vi "ADC SNR_Sweep_working.vi"(8 "error in (no error)":errorcluster, 9 "Sequence parameters":string[][](array[string])=[["Min limit", "Max limit", "Register sheet file", "Register Sheet"], ["", "", "CC2600.xls", "TX_BLE;Trim"], ["Reg write (addr;value)", "Operating frequency [Hz]", "", ""], ["NA", "2.44G", "", ""]], 10 "Run type":i32, 11 "Method parameters":T3={"Dev"={"Do not disturb DUT"=FALSE, "XOSC"=32000000.0, "Board type"="", "EM"="", "Configure tempboard"=TRUE, "Device specific info"=[], "Generic Object"=refnum}, "Method"={"Run type"=1, "Test name"="Current LPM2 4", "Comment"="", "Results folder"="", "AFC"=enum."Off", "Method name"="Current LPM2 4", "Method results"={"Excel brief report"=FALSE, "Spotfire report"=FALSE, "Starfish report"=FALSE}, "Operator"="", "Reference time"=timestamp(0 s since 1904-01-01), "AFC delay"=0.0, "Initialization"=enum."Enabled", "MD5 Sum"="", "HW addon board"=enum."None", "AFC Regsheet"="", "AFC Regfile"=path "", "dummy"=0.0}, "Inst"={"Instr"={"PS1"={"Name"="", "GPIB address"="", "VISA session"=""}, "PS2"={"Name"="", "GPIB address"="", "VISA session"=""}, "TC1"={"Name"="", "GPIB address"="", "VISA session"=""}, "TC2"={"Name"="", "GPIB address"="", "VISA session"=""}, "SA1"={"Name"="", "GPIB address"="", "VISA session"=""}, "SA2"={"Name"="", "GPIB address"="", "VISA session"=""}, "SG1"={"Name"="", "GPIB address"="", "VISA session"=""}, "SG2"={"Name"="", "GPIB address"="", "VISA session"=""}, "SG3"={"Name"="", "GPIB address"="", "VISA session"=""}, "MI1"={"Name"="", "GPIB address"="", "VISA session"=""}, "MI2"={"Name"="", "GPIB address"="", "VISA session"=""}, "SW SA"={"Name"="", "Controller addr"=""}, "SW SG"={"Name"="", "Controller addr"=""}, "MI3"={"Name"="", "GPIB address"="", "VISA session"=""}}, "Switchbox"={"RF Path"=0, "Cal compensation"=enum."TX", "Switchbox gain mode"="", "State"=enum."TX"}, "Instr to control (i.e. SA1)"="Default", "Intrument info string"=""}, "Sequence parameters"=[["Weight", "Min Limit", "Max Limit", "Register Sheet", "", "", "", "", "", "", "", "", ""], ["Vital", "", "1", "LPM2", "", "", "", "", "", "", "", "", ""], ["Resolution", "Reg write (addr;value)", "Chip mode", "Range", "", "", "", "", "", "", "", "", ""], ["u", "NA", "", "auto", "", "", "", "", "", "", "", "", ""]], "Cond"={"Temp logged"=25.0, "VDD1_PS1_6V"=-999.0, "VDD2_PS1_25V"=-999.0, "VDD4_PS2_25V"=-999.0, "VDD3_PS2_6V"=-999.0}, "Meas config"={"X-axis inner loop index"=32000000, "Y-axis outer loop index"=32000000, "X-axis"=[], "Y-axis"=[], "X-axis array req size"=32000000, "Y-axis array req size"=32000000, "Param description"=[], "Use meas clust for reporting"=FALSE, "Parameter index (page)"=0, "X-axis name"="", "Y-axis name"=""}} {"Cond"."VDD3_PS2_6V" format="%.3f"; "Cond"."VDD4_PS2_25V" format="%.3f"; "Cond"."VDD2_PS1_25V" format="%.3f"; "Cond"."VDD1_PS1_6V" format="%.3f"; "Method"."dummy" format="%.1p"; "Method"."AFC delay" format="%.1p"; "Dev"."XOSC" format="%.3p"}) -> (0 "error out":errorcluster, 1 "End method error":T1, 2 "Short Results":string[](array[string]), 3 "Result summary":string[][](array[string])=[["Critical", "Output Power@2405 MHz", "-3", "4", "dBm"], ["Critical", "Output Power@2410 MHz", "-3", "4", "dBm"]])   [LabVIEW 2019]
doc: "[AutoDocStart]Performs crystal accuracy measurements. Measures the offset from ideal frequency. Primarily used for tuning XOSC capacitors and verifying XOSC trims.\n\nSweeping parameters: operating frequency, OSC override value and VDDR level\n\nResults: Offset frequency in ppm[AutoDocEnd]"
uses:
  User Lib/Utilities/Cluster definitions/Method input.ctl
  User Lib/Utilities/Cluster definitions/Device specific info.ctl
  User Lib/Utilities/Controls/Automatic Frequency Compensation types.ctl
  User Lib/Utilities/Controls/Method Reports.ctl
  User Lib/Utilities/Cluster definitions/Method Initialization.ctl
  User Lib/Utilities/Controls/HW addon boards.ctl
  User Lib/Utilities/Cluster definitions/Instr clust.ctl
  User Lib/Utilities/Switchbox control/SwitchBox_State._ENUMctl.ctl
  User Lib/Utilities/Cluster definitions/End method error cluster.ctl
  669fe48b-0ce9-4029-a6ff-6e407436e5b7.vi
  160c279e-5860-4c4e-a522-43dd8a66307b.vi
  470ab757-4a27-4988-8e62-97c7fe5a2084.vi
  56529db9-b118-41d0-9f0e-72512248274d.vi
panel:
  in  "Tab Control":T2(tab)
  # "°C"
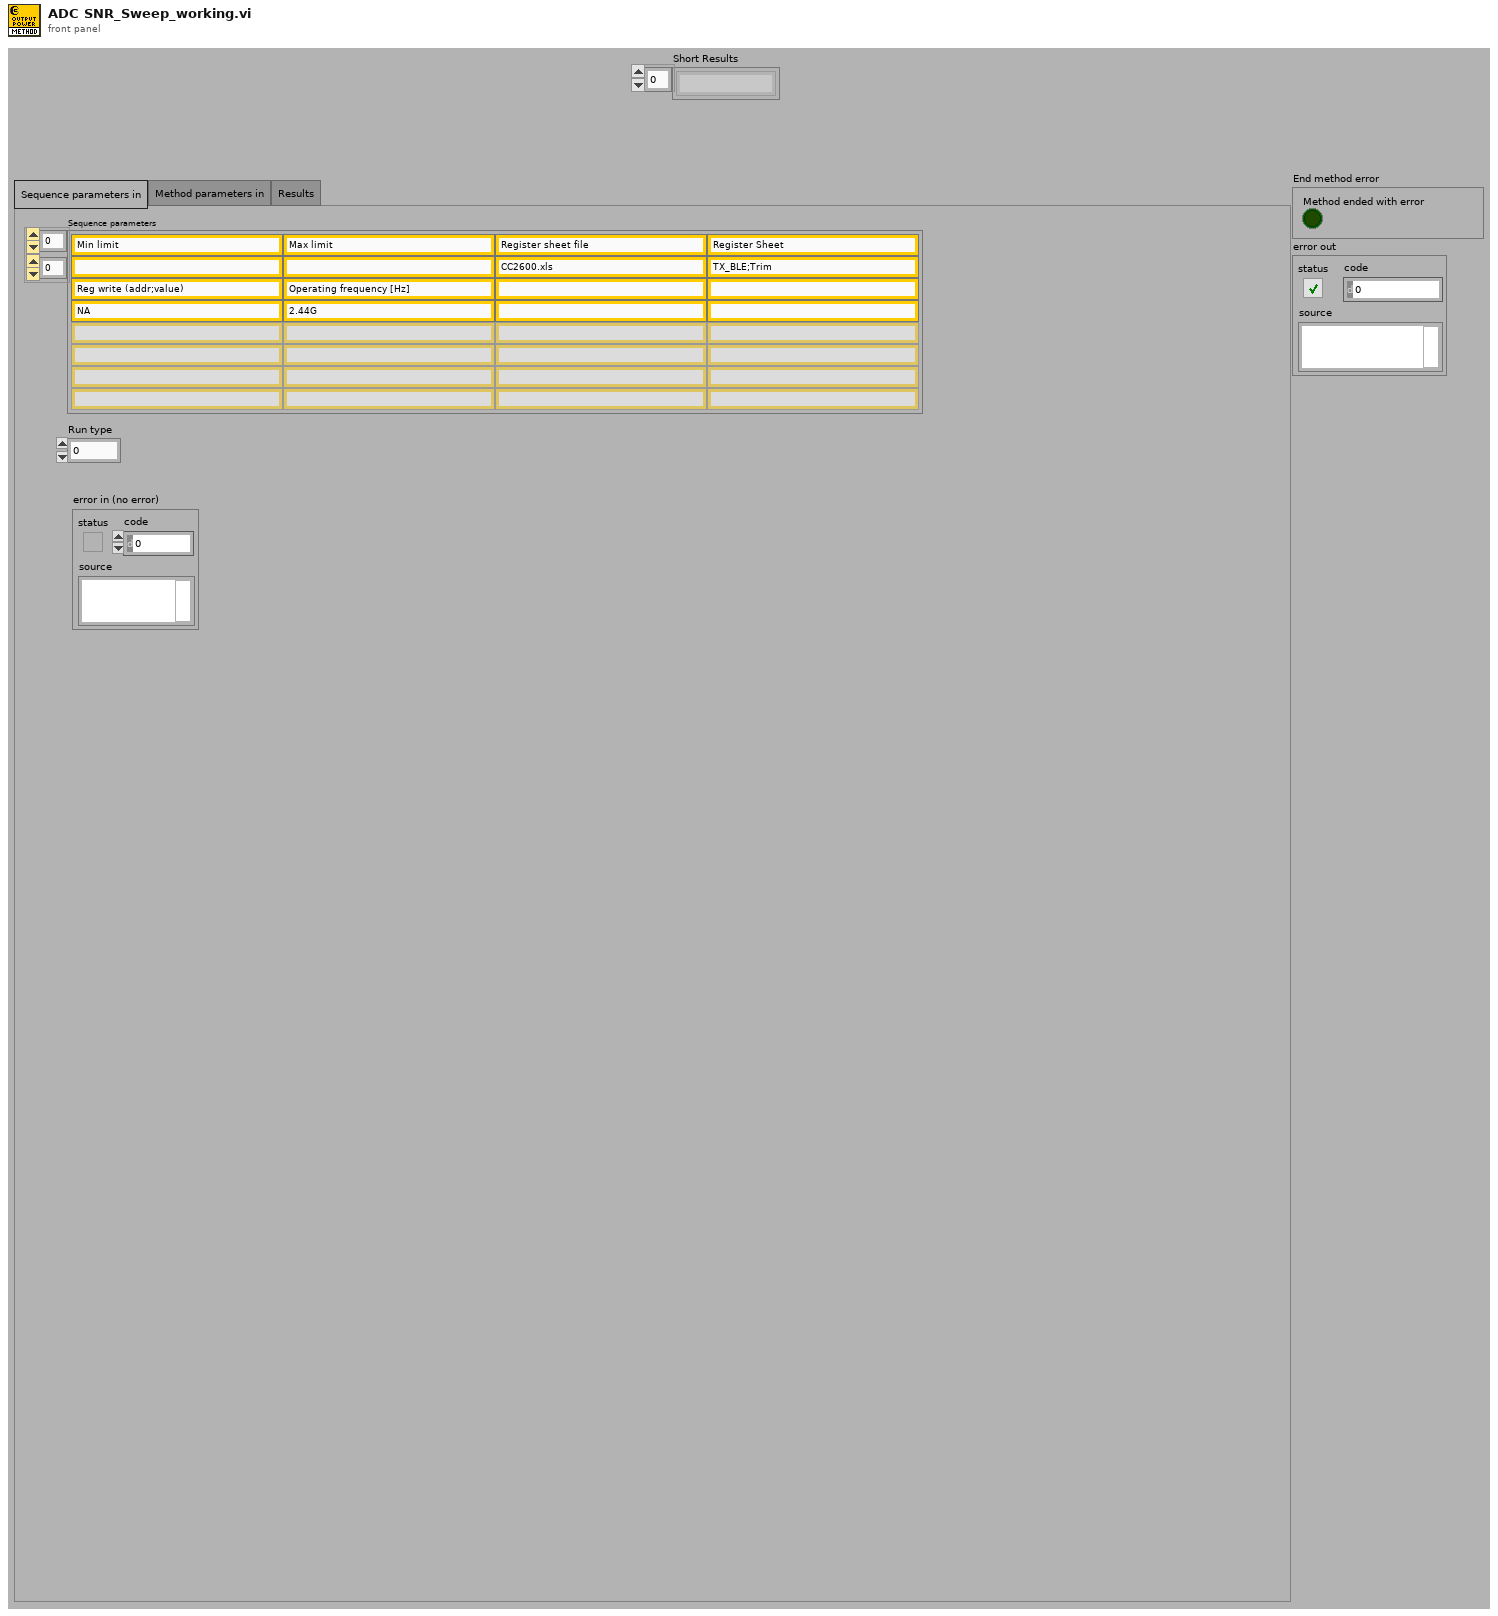
[diagram p1: front panel]
types:
  T1 = typedef "End method error cluster.ctl" = cluster{"Method ended with error":bool}
  T2 = enum32{"Sequence parameters in", "Method parameters in", "Results"}
  T3 = typedef "Method input.ctl" = cluster{"Dev":cluster{"Do not disturb DUT":bool, "XOSC":dbl, "Board type":string, "EM":string, "Configure tempboard":bool, "Device specific info":T4[], "Generic Object":refnum<class>}, "Method":cluster{"Run type":i32, "Test name":string, "Comment":string, "Results folder":string, "AFC":T5, "Method name":string, "Method results":T6, "Operator":string, "Reference time":timestamp, "AFC delay":dbl, "Initialization":T7, "MD5 Sum":string, "HW addon board":T8, "AFC Regsheet":string, "AFC Regfile":path, "dummy":dbl}, "Inst":T9, "Sequence parameters":string[][], "Cond":cluster{"Temp logged":dbl, "VDD1_PS1_6V":dbl, "VDD2_PS1_25V":dbl, "VDD4_PS2_25V":dbl, "VDD3_PS2_6V":dbl}, "Meas config":cluster{"X-axis inner loop index":i32, "Y-axis outer loop index":i32, "X-axis":string[], "Y-axis":string[], "X-axis array req size":i32, "Y-axis array req size":i32, "Param description":string[][], "Use meas clust for reporting":bool, "Parameter index (page)":i32, "X-axis name":string, "Y-axis name":string}}
  T4 = typedef "Device specific info.ctl" = cluster{"EM number":u8, "IP address":string, "Enabled":bool, "Slot no":u8, "RF path":u8, "EM name":string, "Wafer info":string, "AFC frequency ppm":dbl, "Register writes":string[][], "Meas data":string[][][], "Device comment":string}
  T5 = typedef "Automatic Frequency Compensation types.ctl" = enum16{"Off", "Compensate Instrument frequency", "Compensate DUT frequency", "Predictive - Compensate Instrument frequency", "Predictive - Compensate DUT frequency", "Do not skip re-init - Compensate Instrument frequency", "Do not skip re-init - Compensate DUT frequency"}
  T6 = typedef "Method Reports.ctl" = cluster{"Excel brief report":bool, "Spotfire report":bool, "Starfish report":bool}
  T7 = typedef "Method Initialization.ctl" = enum16{"Enabled", "Skip Instr and Device Init", "Enabled with Separate Flash", "Set PS, Device Init and Skip Instr Init", "Skip Device Init"}
  T8 = typedef "HW addon boards.ctl" = enum16{"None", "Current meas 5EM", "Stresstest 10EM"}
  T9 = typedef "Instr clust.ctl" = cluster{"Instr":cluster{"PS1":cluster{"Name":string, "GPIB address":string, "VISA session":refnum<visa-resource-name>}, "PS2":cluster{"Name":string, "GPIB address":string, "VISA session":refnum<visa-resource-name>}, "TC1":cluster{"Name":string, "GPIB address":string, "VISA session":refnum<visa-resource-name>}, "TC2":cluster{"Name":string, "GPIB address":string, "VISA session":refnum<visa-resource-name>}, "SA1":cluster{"Name":string, "GPIB address":string, "VISA session":refnum<visa-resource-name>}, "SA2":cluster{"Name":string, "GPIB address":string, "VISA session":refnum<visa-resource-name>}, "SG1":cluster{"Name":string, "GPIB address":string, "VISA session":refnum<visa-resource-name>}, "SG2":cluster{"Name":string, "GPIB address":string, "VISA session":refnum<visa-resource-name>}, "SG3":cluster{"Name":string, "GPIB address":string, "VISA session":refnum<visa-resource-name>}, "MI1":cluster{"Name":string, "GPIB address":string, "VISA session":refnum<visa-resource-name>}, "MI2":cluster{"Name":string, "GPIB address":string, "VISA session":refnum<visa-resource-name>}, "SW SA":cluster{"Name":string, "Controller addr":string}, "SW SG":cluster{"Name":string, "Controller addr":string}, "MI3":cluster{"Name":string, "GPIB address":string, "VISA session":refnum<visa-resource-name>}}, "Switchbox":cluster{"RF Path":i32, "Cal compensation":enum16{"TX", "RX", "Interferer", "No compensation", "Interferer2"}, "Switchbox gain mode":string, "State":T10}, "Instr to control (i.e. SA1)":string, "Intrument info string":string}
  T10 = typedef "SwitchBox_State._ENUMctl.ctl" = enum16{"TX", "RX", "SP:TX", "SP:RX", "SW:TX", "SW:RX"}
  T11 = cluster{"Fundamental Frequency":dbl, "Sampling Frequncy":dbl, "No of Harmonics":u8, "Window":enum16{"None ", "Hanning", "Hamming", "Blackman-Harris", "Exact Blackman", "Blackman", "Flat Top", "4 Term B-Harris ", "7 Term B-Harris"}, "Blackman (fundamental power) bins)":dbl}
  T12 = enum32{"NI Card Settings", "Memory Read Setting", "DC Capture", "ADC Ramp", "ADC Sine", "SNR", "Cap Calibration"}
  T13 = enum32{"Read from Memory", "Read .dat file", "NI Card Capture", "None"}
  T14 = cluster{"Path to Save plot":path, "Path to Raw Data plot":path}
  T15 = cluster{"Save INL/DNL Plot(Ramp)":bool, "Save SNR Plot":bool, "Save INL/DNL Plot(Sine)":bool, "Save INL/DNL Raw Data(Ramp)":bool, "Save SNR Raw Data":bool, "Save INL/DNL Raw Data(Sine)":bool, "Save DC Raw data":bool, "Save  Raw Data(Sine)":bool}
  T16 = cluster{"SNR":dbl, "SNRD":dbl, "THD":dbl, "ENOB (SNRD)":dbl, "SFDR":dbl, "ENOB (SNR)":dbl, "Noise Power":dbl, "Signal power":dbl}
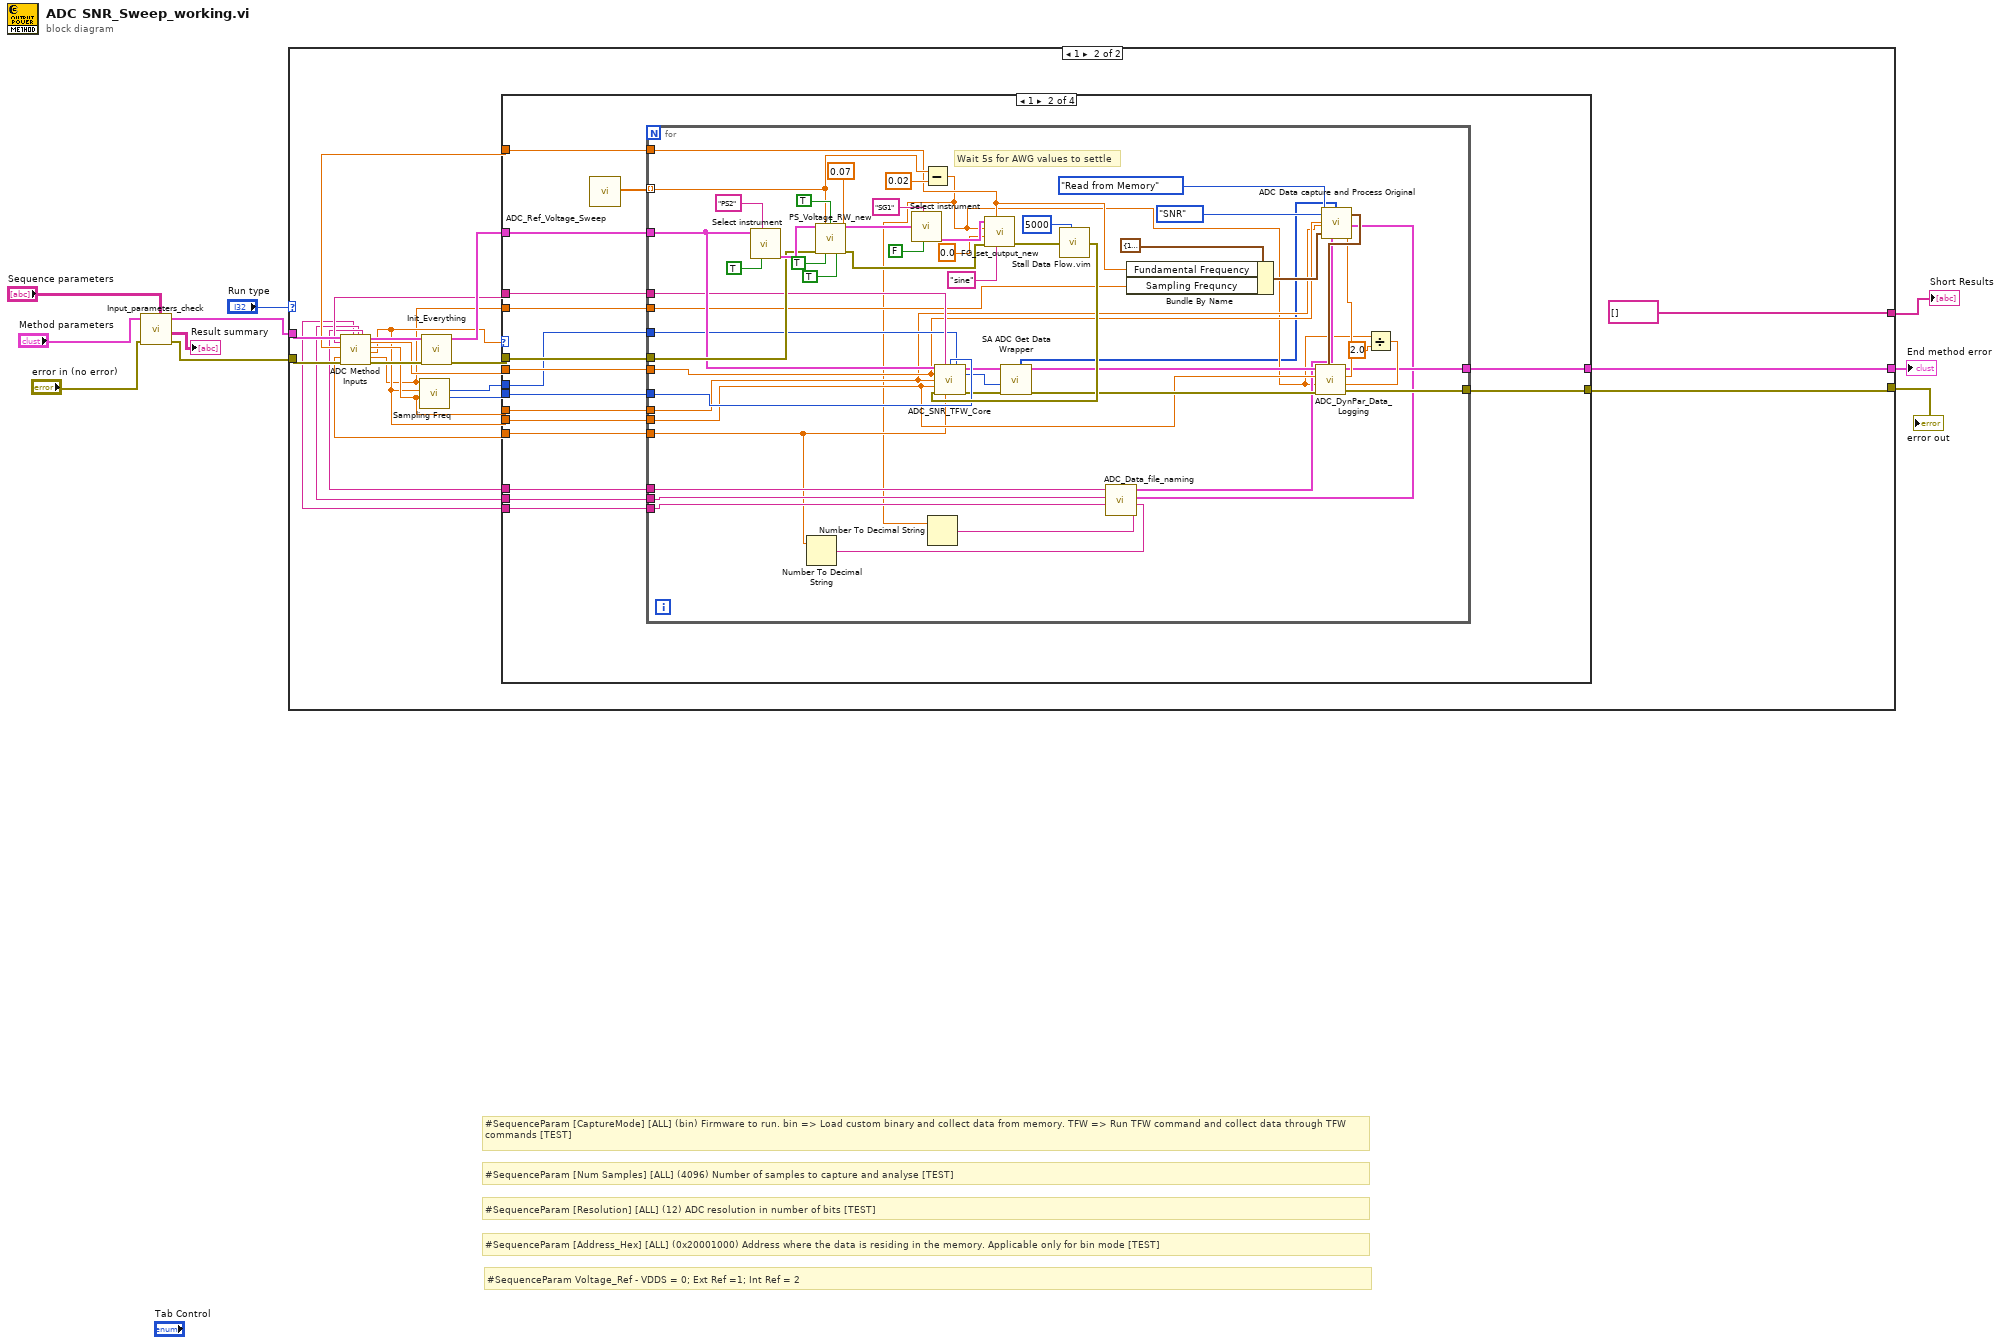
[diagram p0: block diagram]
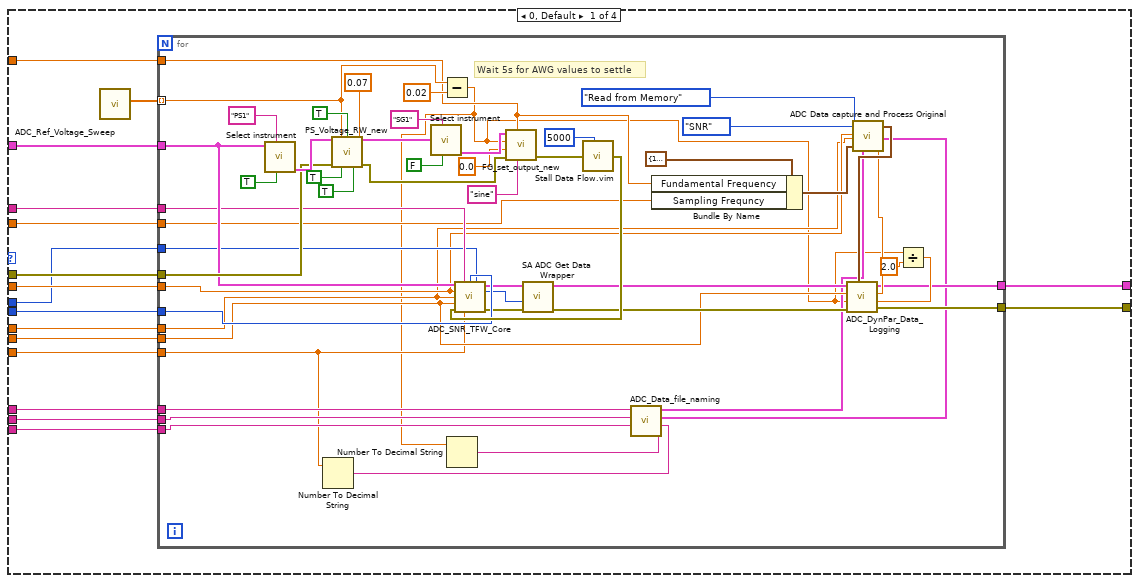
[diagram p3: hidden frame]
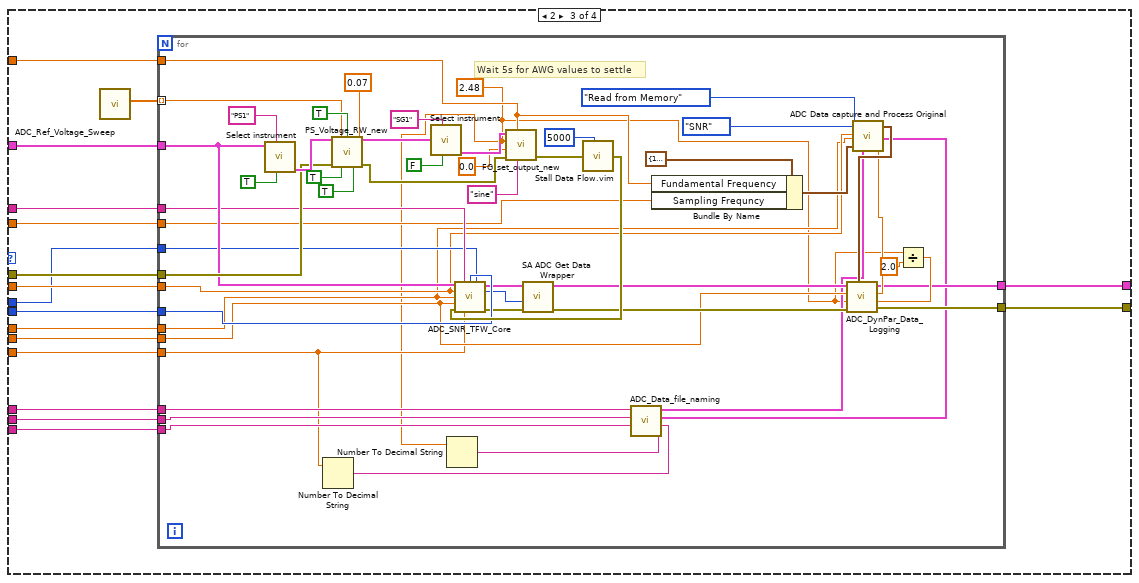
[diagram p4: hidden frame]
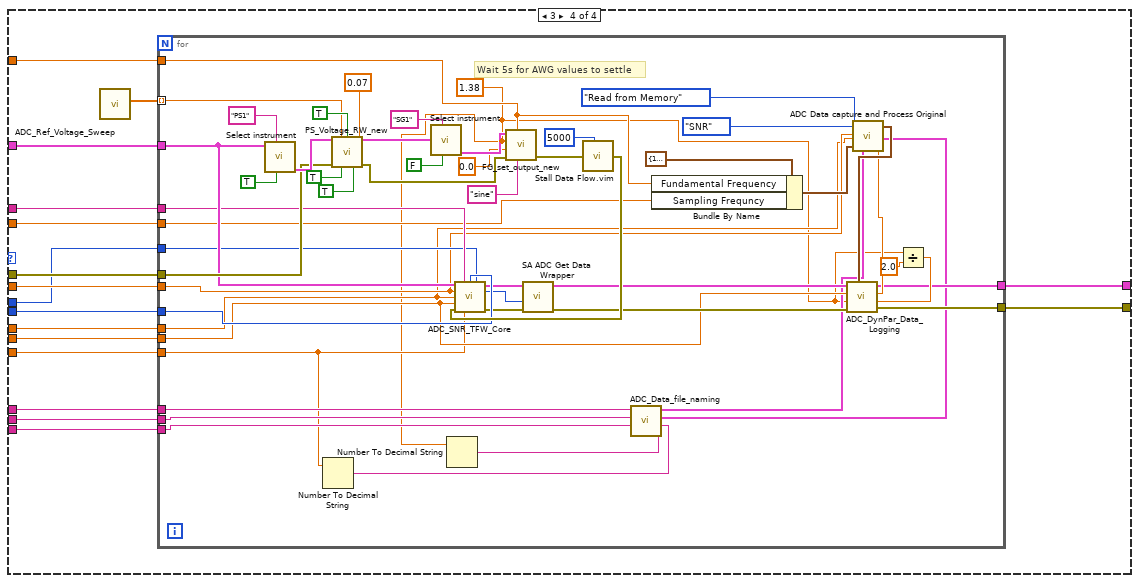
[diagram p5: hidden frame]
diagram:
  # "#SequenceParam Voltage_Ref - VDDS = 0; Ext Ref =1; Int Ref = 2"
  # "#SequenceParam [Num Samples] [ALL] (4096) Number of samples to capture and analyse [TEST]"
  # "#SequenceParam [CaptureMode] [ALL] (bin) Firmware to run. bin => Load custom binary and collect data from memory. TFW => Run TFW command and collect data through TFW commands [TEST]"
  # "#SequenceParam [Address_Hex] [ALL] (0x20001000) Address where the data is residing in the memory. Applicable only for bin mode [TEST]"
  # "#SequenceParam [Resolution] [ALL] (12) ADC resolution in number of bits [TEST]"
  n1 = call "Input_parameters_check.vi"("Sequence parameters"="Sequence parameters", "error in"="error in (no error)", "Method cluster in"="Method parameters") -> ("error out"=w10:errorcluster, "Result summary"=→"Result summary":string[][], "Method cluster out"=w6:T3)  [unwired: 6 in]
  n2 = case shown="1" "Run type" {
    tunnel: w10 -> [w11 w32]
    tunnel: w6 -> [_ w31]
    tunnel: [string[] [] string[] []] -> w3
    tunnel: [w11 w17] -> w2
    tunnel: [_ w16] -> w1
    frame 0, Default {
      # "Run type 0 is only for formatting the result summary"
    }
    frame 1 {
      n3 = call "ADC Method Inputs.vi"("Method cluster in"=w31, "error in (no error)"=w32) -> ("Capture Mode"=w23:string, "Signal Freq"=w20:dbl, "ADC Channel No."=w19:dbl, "Sampling Freq String"=w13:string, "Resolution String"=w14:string, "Voltage Ref String"=w15:string, "Method cluster out"=w30:T3, "Num Samples"=w26:dbl, "Resolution"=w25:dbl, "Voltage Ref"=w24:dbl, "Sampling Freq"=w18:dbl, "error out"=w29:errorcluster)  [unwired: 6 in]
      n4 = call "Sampling Freq.vi"("Resolution"=w25, "Voltage Ref"=w24, "Sampling Freq"=w18) -> ("LGPT Count"=w22:u16, "SCOMP"=w21:u16)  [unwired: 7 in]
      n5 = call "Init_Everything.vi"("error in"=w29, "Method cluster In"=w30) -> ("error out"=w27:errorcluster, "Method cluster out"=w28:T3)  [unwired: 6 in, 2 out]
      n6 = case shown="1" w24 {
        tunnel: w28 -> [w49 w119 w190 w259]
        tunnel: w27 -> [w48 w118 w189 w258]
        tunnel: w26 -> [w47 w117 w188 w257]
        tunnel: w25 -> [w46 w116 w187 w256]
        tunnel: w24 -> [w45 w115 w186 w255]
        tunnel: w23 -> [w44 w114 w185 w254]
        tunnel: w22 -> [w43 w113 w184 w253]
        tunnel: w21 -> [w42 w112 w183 w252]
        tunnel: w20 -> [w41 w111 w182 w251]
        tunnel: w19 -> [w40 w110 w181 w250]
        tunnel: w18 -> [w39 w109 w180 w249]
        tunnel: [w38 w108 w179 w248] -> w16
        tunnel: [w37 w107 w178 w247] -> w17
        tunnel: w15 -> [w36 w106 w177 w246]
        tunnel: w14 -> [w35 w105 w176 w245]
        tunnel: w13 -> [w34 w104 w175 w244]
        frame 0, Default {
          n7 = call "ADC_Ref_Voltage_Sweep.vi"() -> ("Ref voltage sweep"=w50:dbl[])  [unwired: 11 in]
          n8 = for {
            tunnel: w50 -> [w80] mode=indexing
            tunnel: w49 -> [w85]
            tunnel: w48 -> [w87]
            tunnel: w47 -> [w70]
            tunnel: w46 -> [w69]
            tunnel: w45 -> [w64]
            tunnel: w44 -> [w83]
            tunnel: w43 -> [w82]
            tunnel: w42 -> [w81]
            tunnel: w41 -> [w73]
            tunnel: w40 -> [w54]
            tunnel: w39 -> [w72]
            tunnel: [w61] -> w38
            tunnel: [w60] -> w37
            tunnel: w36 -> [w57]
            tunnel: w35 -> [w56]
            tunnel: w34 -> [w55]
            # "Wait 5s for AWG values to settle"
            n9 = call "Select instrument.vi"("Method cluster (T) / Instr cluster (F)"=TRUE, "Instr.Instr to control (i.e. SA1)"="PS1", "Method cluster in"=w85) -> ("Instr out"=w93:T9)  [unwired: 6 in, 2 out]
            n10 = Number To Decimal String(number=w54) -> (decimal integer string=w53:string)  [unwired: 1 in]
            n11 = call "PS_Voltage_RW_new.vi"("InstrCluster in"=w93, "Set Voltage"=w80, "Limit to 4V (T)"=TRUE, "Current(0)"=0.07, "error in (no error)"=w87, "Off (F)                         On (T)"=TRUE, "Read (F)                      Write (T)"=TRUE) -> ("InstrCluster out"=w94:T9, "error out"=w95:errorcluster)  [unwired: 6 in, 1 out]
            n12 = call "Select instrument.vi"("Method cluster (T) / Instr cluster (F)"=FALSE, "Instr.Instr to control (i.e. SA1)"="SG1", "Instr in"=w94) -> ("Instr out"=w98:T9)  [unwired: 6 in, 2 out]
            n13 = Subtract(x=w80, y=0.02) -> (x-y=w52:dbl)
            n14 = Number To Decimal String(number=w52) -> (decimal integer string=w51:string)  [unwired: 1 in]
            n15 = call "FG_set_output_new.vi"("Function (DC, Sine, Square, Triangle, Ramp up, Ramp down, Pulse)"="sine", "Frequency [Hz]"=w73, "error in"=w95, "Low voltage"=0.0, "High voltage (or DC)"=w52, "InstrCluster in"=w98) -> ("error out"=w86:errorcluster)  [unwired: 4 in, 1 out]
            n16 = call "Stall Data Flow.vim"("value in"=w86, "milliseconds to wait"=u32 5000) -> ("value out"=w84:errorcluster)  [unwired: 1 out]
            n17 = call "ADC_SNR_TFW_Core.vi"("Method cluster in"=w85, "Capture Mode"=w83, "LGPT Count"=w82, "SCOMP"=w81, "No. Samples"=w70, "Resolution"=w69, "Voltage Ref"=w64, "error in"=w84, "ADC Chnl No."=w54) -> ("Method cluster out 2"=w78:T3, "ResPar[0] Data Address"=w77:u32, "error out"=w79:errorcluster)  [unwired: 3 in, 1 out]
            n18 = call "SA ADC Get Data Wrapper.vi"("error in"=w79, "Data Address"=w77, "Method cluster in"=w78) -> ("error out"=w66:errorcluster, "output cluster"=w67:T3)  [unwired: 3 in, 4 out]
            n19 = call "ADC_Data_file_naming.vi"("Amplitude (Vpp)"=w51, "ADC Chn. No"=w53, "Sampling Freq String"=w55, "Resolution String"=w56, "Voltage Ref String"=w57) -> ("path to save"=w58:T14, "Save data"=w59:T15)  [unwired: 5 in]
            n20 = Bundle By Name(cluster=T11 {"Fundamental Frequency"=10000.0, "Sampling Frequncy"=250000.0, "No of Harmonics"=9, "Window"=enum."7 Term B-Harris", "Blackman (fundamental power) bins)"=1.0} ("Inputs for Dyanmic para"), "Fundamental Frequency"=w73, "Sampling Frequncy"=w72) -> (w71:T11)
            n21 = call "ADC Data capture and Process Original.vi"("ADC Output Read Method"=T13."Read from Memory", "Select the Tab to project"=T12."SNR", "No.of samples(SNR)"=w70, "Resolution"=w69, "Inputs for Dyanmic para"=w71, "Save data"=w59, "path to save"=w58) -> ("detected Throughput"=w65:dbl, "Dynamic Parameters"=w68:T16)  [unwired: 14 in, 5 out]
            n22 = Divide(x=w52, y=2.0) -> (x/y=w62:dbl)
            n23 = call "ADC_DynPar_Data_Logging.vi"("Offset (V)"=w62, "detected Throughput"=w65, "Dynamic Parameters"=w68, "error in (no error)"=w66, "Amplitude (Vpp)"=w52, "Ref Voltage"=w64, "Method Cluster In"=w67) -> ("error out"=w60:errorcluster, "End method error"=w61:T1)  [unwired: 3 in]
          }
        }
        frame 1 {
          n24 = call "ADC_Ref_Voltage_Sweep.vi"() -> ("Ref voltage sweep"=w120:dbl[])  [unwired: 11 in]
          n25 = for {
            tunnel: w120 -> [w151] mode=indexing
            tunnel: w119 -> [w156]
            tunnel: w118 -> [w158]
            tunnel: w117 -> [w141]
            tunnel: w116 -> [w140]
            tunnel: w115 -> [w135]
            tunnel: w114 -> [w154]
            tunnel: w113 -> [w153]
            tunnel: w112 -> [w152]
            tunnel: w111 -> [w144]
            tunnel: w110 -> [w125]
            tunnel: w109 -> [w143]
            tunnel: [w132] -> w108
            tunnel: [w131] -> w107
            tunnel: w106 -> [w128]
            tunnel: w105 -> [w127]
            tunnel: w104 -> [w126]
            # "Wait 5s for AWG values to settle"
            n26 = call "Select instrument.vi"("Method cluster (T) / Instr cluster (F)"=TRUE, "Instr.Instr to control (i.e. SA1)"="PS2", "Method cluster in"=w156) -> ("Instr out"=w164:T9)  [unwired: 6 in, 2 out]
            n27 = Number To Decimal String(number=w125) -> (decimal integer string=w124:string)  [unwired: 1 in]
            n28 = call "PS_Voltage_RW_new.vi"("InstrCluster in"=w164, "Set Voltage"=w151, "Limit to 4V (T)"=TRUE, "Current(0)"=0.07, "error in (no error)"=w158, "Off (F)                         On (T)"=TRUE, "Read (F)                      Write (T)"=TRUE) -> ("InstrCluster out"=w165:T9, "error out"=w166:errorcluster)  [unwired: 6 in, 1 out]
            n29 = call "Select instrument.vi"("Method cluster (T) / Instr cluster (F)"=FALSE, "Instr.Instr to control (i.e. SA1)"="SG1", "Instr in"=w165) -> ("Instr out"=w169:T9)  [unwired: 6 in, 2 out]
            n30 = Subtract(x=w151, y=0.02) -> (x-y=w123:dbl)
            n31 = Number To Decimal String(number=w123) -> (decimal integer string=w122:string)  [unwired: 1 in]
            n32 = call "FG_set_output_new.vi"("Function (DC, Sine, Square, Triangle, Ramp up, Ramp down, Pulse)"="sine", "Frequency [Hz]"=w144, "error in"=w166, "Low voltage"=0.0, "High voltage (or DC)"=w123, "InstrCluster in"=w169) -> ("error out"=w157:errorcluster)  [unwired: 4 in, 1 out]
            n33 = call "Stall Data Flow.vim"("value in"=w157, "milliseconds to wait"=u32 5000) -> ("value out"=w155:errorcluster)  [unwired: 1 out]
            n34 = call "ADC_SNR_TFW_Core.vi"("Method cluster in"=w156, "Capture Mode"=w154, "LGPT Count"=w153, "SCOMP"=w152, "No. Samples"=w141, "Resolution"=w140, "Voltage Ref"=w135, "error in"=w155, "ADC Chnl No."=w125) -> ("Method cluster out 2"=w149:T3, "ResPar[0] Data Address"=w148:u32, "error out"=w150:errorcluster)  [unwired: 3 in, 1 out]
            n35 = call "SA ADC Get Data Wrapper.vi"("error in"=w150, "Data Address"=w148, "Method cluster in"=w149) -> ("error out"=w137:errorcluster, "output cluster"=w138:T3, "ADC samples"=w121:u32[])  [unwired: 3 in, 3 out]
            n36 = call "ADC_Data_file_naming.vi"("Amplitude (Vpp)"=w122, "ADC Chn. No"=w124, "Sampling Freq String"=w126, "Resolution String"=w127, "Voltage Ref String"=w128) -> ("path to save"=w129:T14, "Save data"=w130:T15)  [unwired: 5 in]
            n37 = Bundle By Name(cluster=T11 {"Fundamental Frequency"=10000.0, "Sampling Frequncy"=250000.0, "No of Harmonics"=9, "Window"=enum."7 Term B-Harris", "Blackman (fundamental power) bins)"=1.0} ("Inputs for Dyanmic para"), "Fundamental Frequency"=w144, "Sampling Frequncy"=w143) -> (w142:T11)
            n38 = call "ADC Data capture and Process Original.vi"("ADC Output Read Method"=T13."Read from Memory", "Select the Tab to project"=T12."SNR", "No.of samples(SNR)"=w141, "Resolution"=w140, "Inputs for Dyanmic para"=w142, "Save data"=w130, "Waveform"=w121, "path to save"=w129) -> ("detected Throughput"=w136:dbl, "Dynamic Parameters"=w139:T16)  [unwired: 13 in, 5 out]
            n39 = Divide(x=w123, y=2.0) -> (x/y=w133:dbl)
            n40 = call "ADC_DynPar_Data_Logging.vi"("Offset (V)"=w133, "detected Throughput"=w136, "Dynamic Parameters"=w139, "error in (no error)"=w137, "Amplitude (Vpp)"=w123, "Ref Voltage"=w135, "Method Cluster In"=w138) -> ("error out"=w131:errorcluster, "End method error"=w132:T1)  [unwired: 3 in]
          }
        }
        frame 2 {
          n41 = call "ADC_Ref_Voltage_Sweep.vi"() -> ("Ref voltage sweep"=w191:dbl[])  [unwired: 11 in]
          n42 = for {
            tunnel: w191 -> [w221] mode=indexing
            tunnel: w190 -> [w226]
            tunnel: w189 -> [w228]
            tunnel: w188 -> [w211]
            tunnel: w187 -> [w210]
            tunnel: w186 -> [w205]
            tunnel: w185 -> [w224]
            tunnel: w184 -> [w223]
            tunnel: w183 -> [w222]
            tunnel: w182 -> [w214]
            tunnel: w181 -> [w195]
            tunnel: w180 -> [w213]
            tunnel: [w202] -> w179
            tunnel: [w201] -> w178
            tunnel: w177 -> [w198]
            tunnel: w176 -> [w197]
            tunnel: w175 -> [w196]
            w192 = 2.48 ("High voltage (or DC)")
            # "Wait 5s for AWG values to settle"
            n43 = call "Select instrument.vi"("Method cluster (T) / Instr cluster (F)"=TRUE, "Instr.Instr to control (i.e. SA1)"="PS1", "Method cluster in"=w226) -> ("Instr out"=w234:T9)  [unwired: 6 in, 2 out]
            n44 = Number To Decimal String(number=w195) -> (decimal integer string=w194:string)  [unwired: 1 in]
            n45 = call "PS_Voltage_RW_new.vi"("InstrCluster in"=w234, "Set Voltage"=w221, "Limit to 4V (T)"=TRUE, "Current(0)"=0.07, "error in (no error)"=w228, "Off (F)                         On (T)"=TRUE, "Read (F)                      Write (T)"=TRUE) -> ("InstrCluster out"=w235:T9, "error out"=w236:errorcluster)  [unwired: 6 in, 1 out]
            n46 = call "Select instrument.vi"("Method cluster (T) / Instr cluster (F)"=FALSE, "Instr.Instr to control (i.e. SA1)"="SG1", "Instr in"=w235) -> ("Instr out"=w239:T9)  [unwired: 6 in, 2 out]
            n47 = Number To Decimal String(number=w192) -> (decimal integer string=w193:string)  [unwired: 1 in]
            n48 = call "FG_set_output_new.vi"("Function (DC, Sine, Square, Triangle, Ramp up, Ramp down, Pulse)"="sine", "Frequency [Hz]"=w214, "error in"=w236, "Low voltage"=0.0, "High voltage (or DC)"=w192, "InstrCluster in"=w239) -> ("error out"=w227:errorcluster)  [unwired: 4 in, 1 out]
            n49 = call "Stall Data Flow.vim"("value in"=w227, "milliseconds to wait"=u32 5000) -> ("value out"=w225:errorcluster)  [unwired: 1 out]
            n50 = call "ADC_SNR_TFW_Core.vi"("Method cluster in"=w226, "Capture Mode"=w224, "LGPT Count"=w223, "SCOMP"=w222, "No. Samples"=w211, "Resolution"=w210, "Voltage Ref"=w205, "error in"=w225, "ADC Chnl No."=w195) -> ("Method cluster out 2"=w219:T3, "ResPar[0] Data Address"=w218:u32, "error out"=w220:errorcluster)  [unwired: 3 in, 1 out]
            n51 = call "SA ADC Get Data Wrapper.vi"("error in"=w220, "Data Address"=w218, "Method cluster in"=w219) -> ("error out"=w207:errorcluster, "output cluster"=w208:T3)  [unwired: 3 in, 4 out]
            n52 = call "ADC_Data_file_naming.vi"("Amplitude (Vpp)"=w193, "ADC Chn. No"=w194, "Sampling Freq String"=w196, "Resolution String"=w197, "Voltage Ref String"=w198) -> ("path to save"=w199:T14, "Save data"=w200:T15)  [unwired: 5 in]
            n53 = Bundle By Name(cluster=T11 {"Fundamental Frequency"=10000.0, "Sampling Frequncy"=250000.0, "No of Harmonics"=9, "Window"=enum."7 Term B-Harris", "Blackman (fundamental power) bins)"=1.0} ("Inputs for Dyanmic para"), "Fundamental Frequency"=w214, "Sampling Frequncy"=w213) -> (w212:T11)
            n54 = call "ADC Data capture and Process Original.vi"("ADC Output Read Method"=T13."Read from Memory", "Select the Tab to project"=T12."SNR", "No.of samples(SNR)"=w211, "Resolution"=w210, "Inputs for Dyanmic para"=w212, "Save data"=w200, "path to save"=w199) -> ("detected Throughput"=w206:dbl, "Dynamic Parameters"=w209:T16)  [unwired: 14 in, 5 out]
            n55 = Divide(x=w192, y=2.0) -> (x/y=w203:dbl)
            n56 = call "ADC_DynPar_Data_Logging.vi"("Offset (V)"=w203, "detected Throughput"=w206, "Dynamic Parameters"=w209, "error in (no error)"=w207, "Amplitude (Vpp)"=w192, "Ref Voltage"=w205, "Method Cluster In"=w208) -> ("error out"=w201:errorcluster, "End method error"=w202:T1)  [unwired: 3 in]
          }
        }
        frame 3 {
          n57 = call "ADC_Ref_Voltage_Sweep.vi"() -> ("Ref voltage sweep"=w260:dbl[])  [unwired: 11 in]
          n58 = for {
            tunnel: w260 -> [w290] mode=indexing
            tunnel: w259 -> [w295]
            tunnel: w258 -> [w297]
            tunnel: w257 -> [w280]
            tunnel: w256 -> [w279]
            tunnel: w255 -> [w274]
            tunnel: w254 -> [w293]
            tunnel: w253 -> [w292]
            tunnel: w252 -> [w291]
            tunnel: w251 -> [w283]
            tunnel: w250 -> [w264]
            tunnel: w249 -> [w282]
            tunnel: [w271] -> w248
            tunnel: [w270] -> w247
            tunnel: w246 -> [w267]
            tunnel: w245 -> [w266]
            tunnel: w244 -> [w265]
            w261 = 1.38 ("High voltage (or DC)")
            # "Wait 5s for AWG values to settle"
            n59 = call "Select instrument.vi"("Method cluster (T) / Instr cluster (F)"=TRUE, "Instr.Instr to control (i.e. SA1)"="PS1", "Method cluster in"=w295) -> ("Instr out"=w303:T9)  [unwired: 6 in, 2 out]
            n60 = Number To Decimal String(number=w264) -> (decimal integer string=w263:string)  [unwired: 1 in]
            n61 = call "PS_Voltage_RW_new.vi"("InstrCluster in"=w303, "Set Voltage"=w290, "Limit to 4V (T)"=TRUE, "Current(0)"=0.07, "error in (no error)"=w297, "Off (F)                         On (T)"=TRUE, "Read (F)                      Write (T)"=TRUE) -> ("InstrCluster out"=w304:T9, "error out"=w305:errorcluster)  [unwired: 6 in, 1 out]
            n62 = call "Select instrument.vi"("Method cluster (T) / Instr cluster (F)"=FALSE, "Instr.Instr to control (i.e. SA1)"="SG1", "Instr in"=w304) -> ("Instr out"=w308:T9)  [unwired: 6 in, 2 out]
            n63 = Number To Decimal String(number=w261) -> (decimal integer string=w262:string)  [unwired: 1 in]
            n64 = call "FG_set_output_new.vi"("Function (DC, Sine, Square, Triangle, Ramp up, Ramp down, Pulse)"="sine", "Frequency [Hz]"=w283, "error in"=w305, "Low voltage"=0.0, "High voltage (or DC)"=w261, "InstrCluster in"=w308) -> ("error out"=w296:errorcluster)  [unwired: 4 in, 1 out]
            n65 = call "Stall Data Flow.vim"("value in"=w296, "milliseconds to wait"=u32 5000) -> ("value out"=w294:errorcluster)  [unwired: 1 out]
            n66 = call "ADC_SNR_TFW_Core.vi"("Method cluster in"=w295, "Capture Mode"=w293, "LGPT Count"=w292, "SCOMP"=w291, "No. Samples"=w280, "Resolution"=w279, "Voltage Ref"=w274, "error in"=w294, "ADC Chnl No."=w264) -> ("Method cluster out 2"=w288:T3, "ResPar[0] Data Address"=w287:u32, "error out"=w289:errorcluster)  [unwired: 3 in, 1 out]
            n67 = call "SA ADC Get Data Wrapper.vi"("error in"=w289, "Data Address"=w287, "Method cluster in"=w288) -> ("error out"=w276:errorcluster, "output cluster"=w277:T3)  [unwired: 3 in, 4 out]
            n68 = call "ADC_Data_file_naming.vi"("Amplitude (Vpp)"=w262, "ADC Chn. No"=w263, "Sampling Freq String"=w265, "Resolution String"=w266, "Voltage Ref String"=w267) -> ("path to save"=w268:T14, "Save data"=w269:T15)  [unwired: 5 in]
            n69 = Bundle By Name(cluster=T11 {"Fundamental Frequency"=10000.0, "Sampling Frequncy"=250000.0, "No of Harmonics"=9, "Window"=enum."7 Term B-Harris", "Blackman (fundamental power) bins)"=1.0} ("Inputs for Dyanmic para"), "Fundamental Frequency"=w283, "Sampling Frequncy"=w282) -> (w281:T11)
            n70 = call "ADC Data capture and Process Original.vi"("ADC Output Read Method"=T13."Read from Memory", "Select the Tab to project"=T12."SNR", "No.of samples(SNR)"=w280, "Resolution"=w279, "Inputs for Dyanmic para"=w281, "Save data"=w269, "path to save"=w268) -> ("detected Throughput"=w275:dbl, "Dynamic Parameters"=w278:T16)  [unwired: 14 in, 5 out]
            n71 = Divide(x=w261, y=2.0) -> (x/y=w272:dbl)
            n72 = call "ADC_DynPar_Data_Logging.vi"("Offset (V)"=w272, "detected Throughput"=w275, "Dynamic Parameters"=w278, "error in (no error)"=w276, "Amplitude (Vpp)"=w261, "Ref Voltage"=w274, "Method Cluster In"=w277) -> ("error out"=w270:errorcluster, "End method error"=w271:T1)  [unwired: 3 in]
          }
        }
      }
    }
  }
  "Short Results" <- w3
  "End method error" <- w1
  "error out" <- w2
